vi "Load Numeric Keypad.vi"(4 "Password":bool, 6 "Divide":dbl=1.0, 7 "Show Value Initially":bool, 8 "error in (no error)":errorcluster, 9 "Initial Value":dbl, 10 "Numeric ctrlRef":refnum<vi>, 11 "VI Refnum":refnum<vi>) -> (0 "error out":errorcluster)   [LabVIEW 2014]
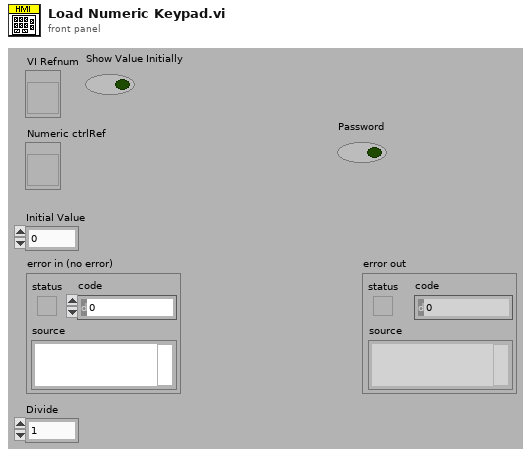
[diagram p1: front panel]
types:
  T1 = enum32{"Bad", "Idle", "Run top level", "Running"}
  T2 = enum32{"Invalid", "Standard", "Closed", "Hidden", "Minimized", "Maximized"}
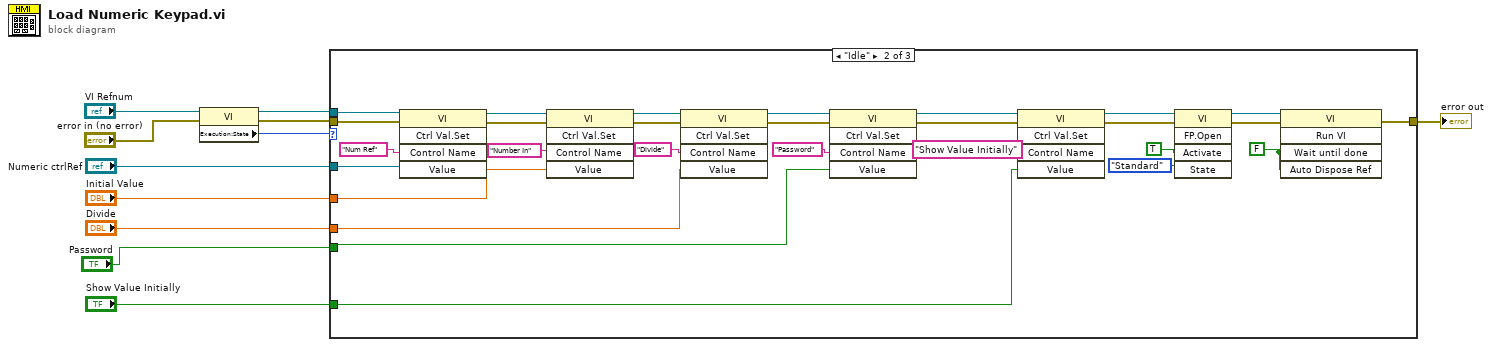
[diagram p0: block diagram]
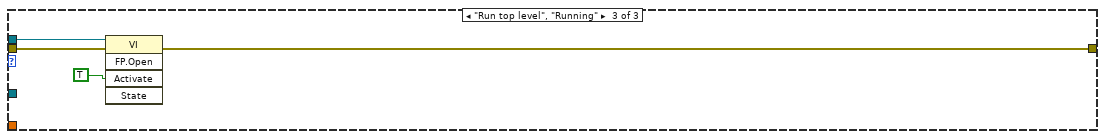
[diagram p3: hidden frame]
diagram:
  n1 = property class="VI"(reference="VI Refnum", error in="error in (no error)") -> (reference out=w10:refnum<vi>, error out=w9:errorcluster, "Execution:State"=w11:T1)
  n2 = case shown="\"Idle\"" w11 {
    tunnel: w10 -> [_ w38 w43]
    tunnel: w9 -> [w12 w40 w42]
    tunnel: "Initial Value" -> [_ w29 _]
    tunnel: "Numeric ctrlRef" -> [_ w25 _]
    tunnel: "Divide" -> [_ w24 _]
    tunnel: [w12 w23 w41] -> w3
    tunnel: "Password" -> [_ w19 _]
    tunnel: "Show Value Initially" -> [_ w14 _]
    frame "Bad", Default {
    }
    frame "Idle" {
      w37 = FALSE ("Wait until done")
      n3 = invoke class="VI" method="Ctrl Val.Set"(reference=w38, error in=w40, "Control Name"="Num Ref", "Value"=w25) -> (reference out=w32:refnum<vi>, error out=w31:errorcluster)  [unwired: 1 in, 3 out]
      n4 = invoke class="VI" method="Ctrl Val.Set"(reference=w32, error in=w31, "Control Name"="Number In", "Value"=w29) -> (reference out=w27:refnum<vi>, error out=w26:errorcluster)  [unwired: 1 in, 3 out]
      n5 = invoke class="VI" method="Ctrl Val.Set"(reference=w27, error in=w26, "Control Name"="Divide", "Value"=w24) -> (reference out=w22:refnum<vi>, error out=w21:errorcluster)  [unwired: 1 in, 3 out]
      n6 = invoke class="VI" method="Ctrl Val.Set"(reference=w22, error in=w21, "Control Name"="Password", "Value"=w19) -> (reference out=w18:refnum<vi>, error out=w17:errorcluster)  [unwired: 1 in, 3 out]
      n7 = invoke class="VI" method="Ctrl Val.Set"(reference=w18, error in=w17, "Control Name"="Show Value Initially", "Value"=w14) -> (reference out=w16:refnum<vi>, error out=w15:errorcluster)  [unwired: 1 in, 3 out]
      n8 = invoke class="VI" method="FP.Open"(reference=w16, error in=w15, "Activate"=TRUE, "State"=T2."Standard") -> (reference out=w34:refnum<vi>, error out=w33:errorcluster)  [unwired: 1 in, 3 out]
      n9 = invoke class="VI" method="Run VI"(reference=w34, error in=w33, "Wait until done"=w37, "Auto Dispose Ref"=w37) -> (error out=w23:errorcluster)  [unwired: 1 in, 4 out]
    }
    frame "Run top level", "Running" {
      n10 = invoke class="VI" method="FP.Open"(reference=w43, error in=w42, "Activate"=TRUE) -> (error out=w41:errorcluster)  [unwired: 2 in, 4 out]
    }
  }
  "error out" <- w3
